vi "ManualControlExitCheck.vi"(10 "Stop Switch":T1={"Tag Name"="S060.PXI.Signals.PlltData.SN", "Network Path"="172.15.51.1,1,0", "use opc"=FALSE, "DataSocket Reference"={"CWDSLib._DCWDataSocket"=refnum, "CWDSLib._DCWData"=refnum, "OnDataUpdated"=0, "OnStatusUpdated"=0}} {"DataSocket Reference"."OnStatusUpdated" format="%.0x"; "DataSocket Reference"."OnDataUpdated" format="%.0x"}, 11 "Action Switch":T1={"Tag Name"="S060.PXI.Signals.PlltData.SN", "Network Path"="172.15.51.1,1,0", "use opc"=FALSE, "DataSocket Reference"={"CWDSLib._DCWDataSocket"=refnum, "CWDSLib._DCWData"=refnum, "OnDataUpdated"=0, "OnStatusUpdated"=0}} {"DataSocket Reference"."OnStatusUpdated" format="%.0x"; "DataSocket Reference"."OnDataUpdated" format="%.0x"}) -> (3 "manual":bool)   [LabVIEW 2018]
uses:
  05.UserVI's/type defs/plc path and tag.ctl
  <vilib>/Platform/dataskt.llb/DataSocket Reference Type.ctl
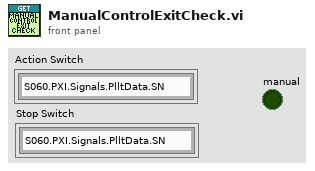
[diagram p1: front panel]
types:
  T1 = typedef "plc path and tag.ctl" = cluster{"Tag Name":string, "Network Path":string, "use opc":bool, "DataSocket Reference":T2}
  T2 = typedef "DataSocket Reference Type.ctl" = cluster{"CWDSLib._DCWDataSocket":refnum<k7>, "CWDSLib._DCWData":refnum<k7>, "OnDataUpdated":u32, "OnStatusUpdated":u32}
  T3 = enum16{"Read SW", "Caculate Time", "SW Release", "Check Stop"}
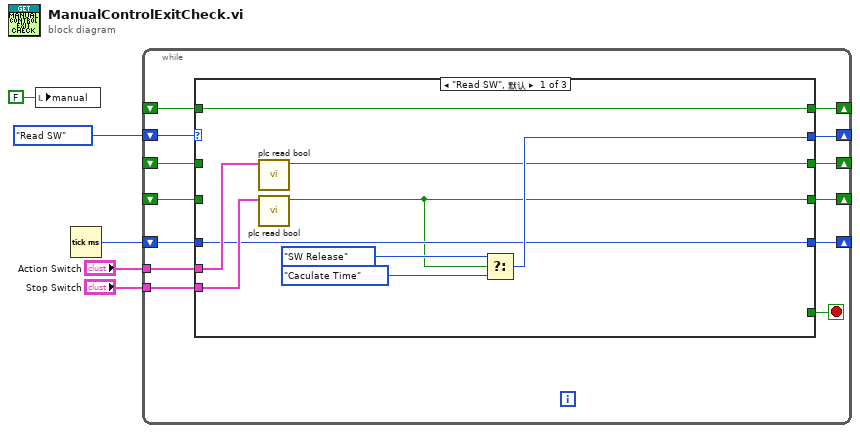
[diagram p0: block diagram]
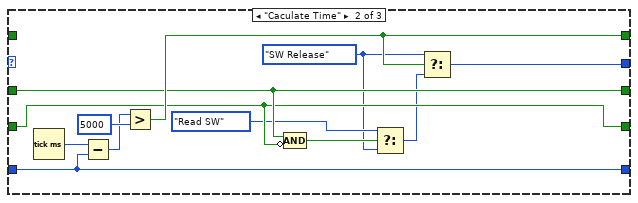
[diagram p2: hidden frame]
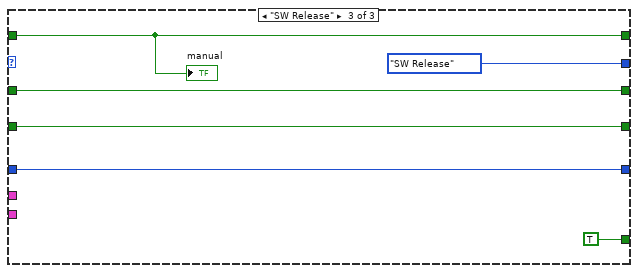
[diagram p3: hidden frame]
diagram:
  n1 = local write "manual"(FALSE) -> ()
  n2 = Tick Count (ms)() -> (millisecond timer value=w4:u32)
  n3 = while {
    shift-right: [w18] -> _
    shift-left: _ -> [w9]
    shift-right: [w17] -> _
    shift-left: _ -> [w8]
    shift-right: [w15] -> _
    shift-left: T3."Read SW" -> [w16]
    shift-right: [w12] -> _
    shift-left: w4 -> [w11]
    tunnel: "Action Switch" -> [w14]
    tunnel: "Stop Switch" -> [w13]
    shift-right: [w10] -> _
    shift-left: _ -> [w6]
    stop <- w7 stop-if-true
    n4 = case shown="\"Read SW\", 默认" w16 {
      tunnel: [w23 w33 w44] -> w18
      tunnel: [w19 w32 w43] -> w17
      tunnel: [w24 w36 T3."SW Release"] -> w15
      tunnel: w14 -> [w27 _ _]
      tunnel: w13 -> [w26 _ _]
      tunnel: [w22 w35 w45] -> w12
      tunnel: w11 -> [w22 w35 w45]
      tunnel: [w21 w34 w41] -> w10
      tunnel: w6 -> [w21 _ w41]
      tunnel: w9 -> [_ w33 w44]
      tunnel: w8 -> [_ w32 w43]
      tunnel: [_ _ TRUE ("value")] -> w7
      frame "Read SW", Default {
        n5 = call "plc read bool.vi"("addr,tag"=w27) -> ("value"=w23:bool)  [unwired: 9 in, 1 out]
        n6 = call "plc read bool.vi"("addr,tag"=w26) -> ("value"=w19:bool)  [unwired: 9 in, 1 out]
        n7 = Select(t=enum16{"Read SW", "Caculate Time", "SW Release"}."SW Release", s=w19, f=enum16{"Read SW", "Caculate Time", "SW Release"}."Caculate Time") -> (s? t:f=w24:enum16{"Read SW", "Caculate Time", "SW Release"})
      }
      frame "Caculate Time" {
        w29 = T3."SW Release"
        n8 = Tick Count (ms)() -> (millisecond timer value=w39:u32)
        n9 = Subtract(x=w39, y=w35) -> (x-y=w37:u32)
        n10 = Greater?(x=w37, y=u32 5000 ("x")) -> (0:w34:bool)
        n11 = Compound Arithmetic op=AND ("复合运算")(w33, invert w32) -> (w31:bool)
        n12 = Select(t=T3."Read SW", s=w31, f=w29) -> (s? t:f=w28:T3)
        n13 = Select(t=w29, s=w34, f=w28) -> (s? t:f=w36:T3)
      }
      frame "SW Release" {
        "manual" <- w41
      }
    }
  }
